vi "showDialog.vi"(0 "HB_TwoButtonDiolog in":refnum<class "HB_TwoButtonDiolog.lvclass">, 11 "error in (no error)":errorcluster) -> (4 "HB_TwoButtonDiolog out":refnum<class "HB_TwoButtonDiolog.lvclass">, 8 "Button Index":i16, 15 "error out":errorcluster)   [LabVIEW 2009, in "HB_Inherance_Example.lvlib" / "HB_TwoButtonDiolog.lvclass"]
doc: "Override VI. This VI implements the display of a two button dialog."
uses:
  HB_TwoButtonDiolog.lvclass
  HB_Dialog/HB_Dialog.lvclass
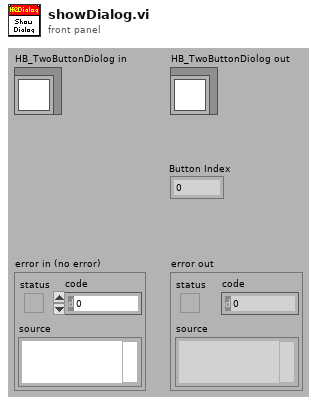
[diagram p1: front panel]
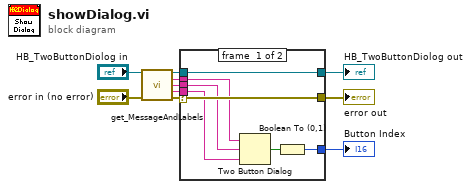
[diagram p0: block diagram]
diagram:
  n1 = call "get_MessageAndLabels.vi"("HB_Dialog in"="HB_TwoButtonDiolog in", "error in (no error)"="error in (no error)") -> ("HB_Dialog out"=w9:refnum<class "HB_TwoButtonDiolog.lvclass">, "Message"=w7:string, "T button name"=w6:string, "F button name"=w5:string, "error out"=w8:errorcluster)  [unwired: 9 in]
  n2 = case shown="No Error" w8 {
    selector: w8 -> [w16 w18]
    tunnel: w7 -> [w14 _]
    tunnel: w6 -> [w13 _]
    tunnel: [w11 _] -> w1
    tunnel: [w16 w18] -> w2
    tunnel: [w15 w19] -> w3
    tunnel: w9 -> [w15 w19]
    tunnel: w5 -> [w12 _]
    frame #0 {
      n3 = Two Button Dialog(message=w14, 1:w12, 2:w13) -> (T button?=w17:bool)
      n4 = Boolean To (0,1)(Boolean=w17) -> (0, 1=w11:i16)
    }
    frame #1 {
    }
  }
  "error out" <- w2
  "HB_TwoButtonDiolog out" <- w3
  "Button Index" <- w1
